vi "Test Acquisition API.vi"() -> ()   [LabVIEW 2026]
doc: "Acquisition API Tester.\n_____\nBased on DQMH Dev Tools: Project Template 7.1.2.1547."
uses:
  <vilib>/Utility/error.llb/DialogType.ctl
  Acquisition.lvlib
  Settings Editor/Settings Editor.lvlib
panel:
  in  "Show Diagram on Init":bool
  in  "Settings":bool
  out "last error":errorcluster
  out "Calibrated?":bool
  in  "Calibrate":bool
  out "Waveform Chart":waveform(dbl)[](graph)
  out "Acquiring?":bool
  in  "Stop Acquiring":bool
  out "HW ID":string
  in  "Start Acquiring":bool
  in  "Show Block Diagram":bool
  in  "Stop Module":bool
  in  "Start Module":bool
  in  "Hide Module Panel":bool
  in  "Show Module Panel":bool
  out "Status":string
  out "Module Running?":bool
  # "This VI tests the API for the Module."
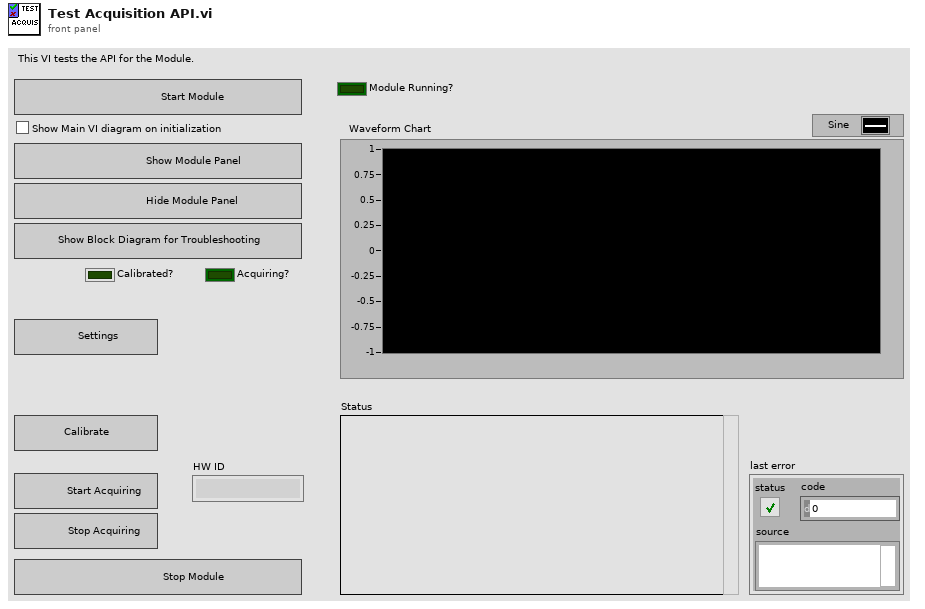
[diagram p1: front panel]
types:
  T1 = typedef "Acquisition.lvlib/Broadcast Events--cluster.ctl" = cluster{"Module Did Init":refnum<user-event>, "Status Updated":refnum<user-event>, "Error Reported":refnum<user-event>, "Module Did Stop":refnum<user-event>, "Update Module Execution Status":refnum<user-event>, "Acquisition Started":refnum<user-event>, "Acquisition Stopped":refnum<user-event>, "Data Updated":refnum<user-event>, "Device Calibrated":refnum<user-event>}
  T2 = typedef "DialogType.ctl" = u16
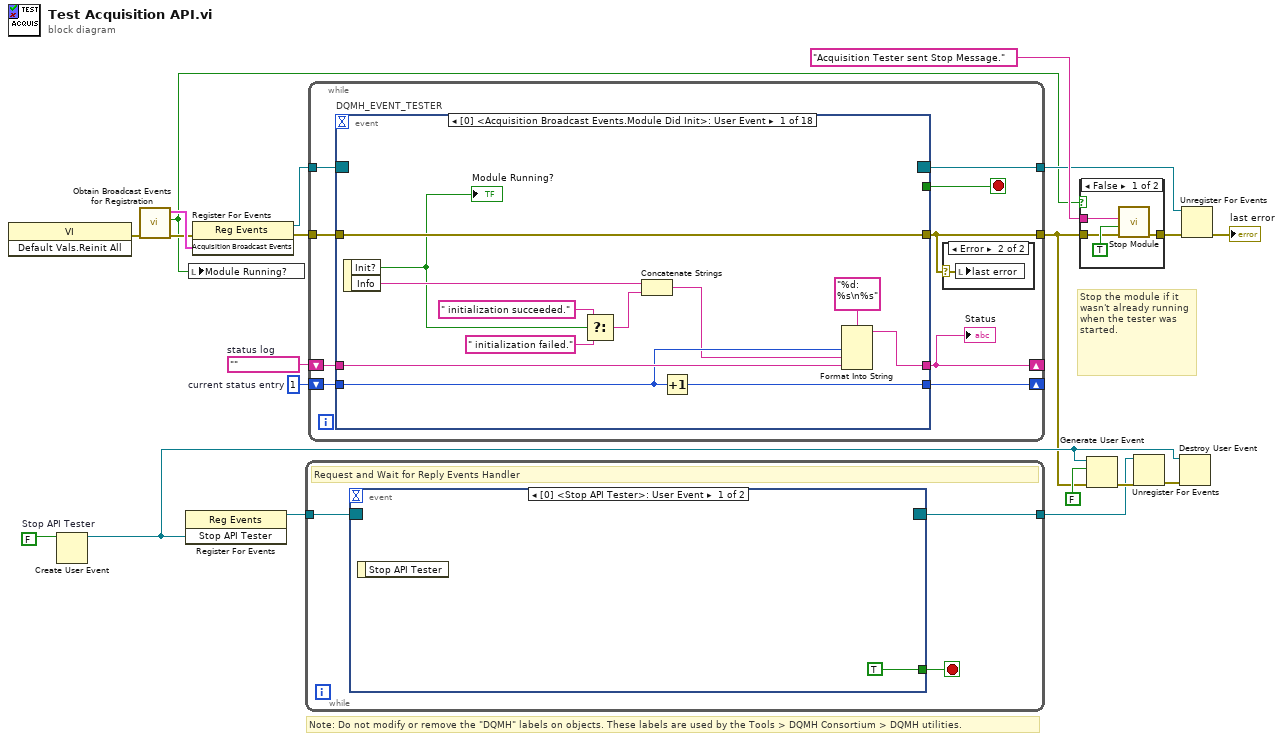
[diagram p0: block diagram]
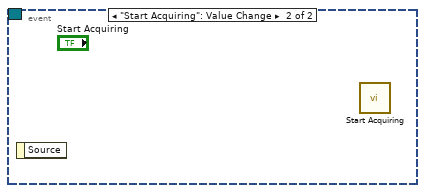
[diagram p2: hidden frame]
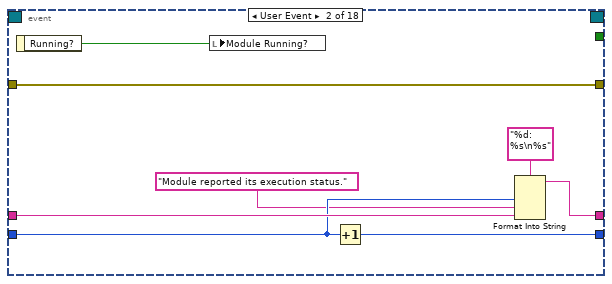
[diagram p4: hidden frame]
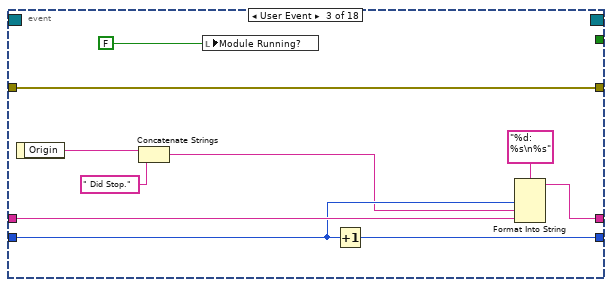
[diagram p5: hidden frame]
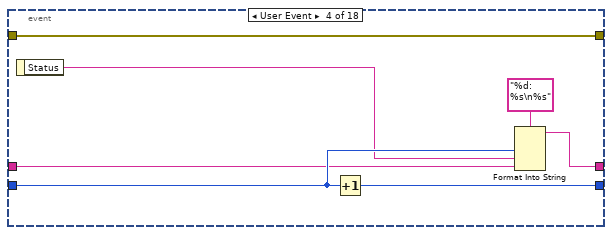
[diagram p6: hidden frame]
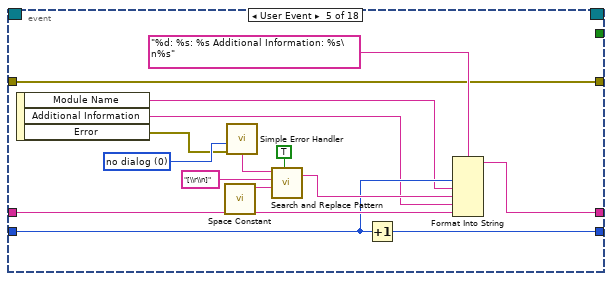
[diagram p7: hidden frame]
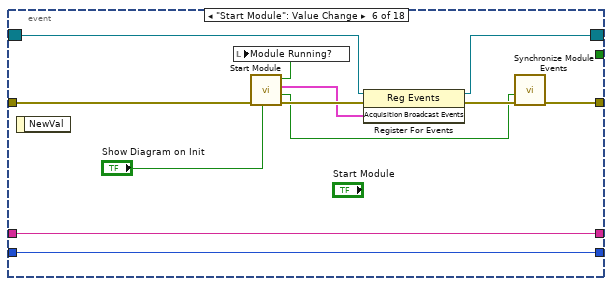
[diagram p8: hidden frame]
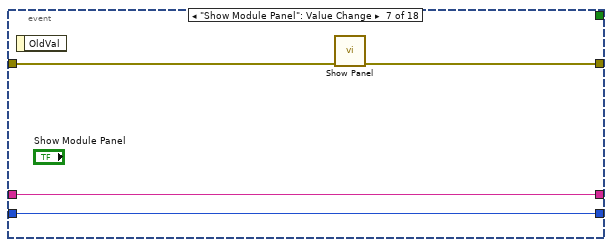
[diagram p9: hidden frame]
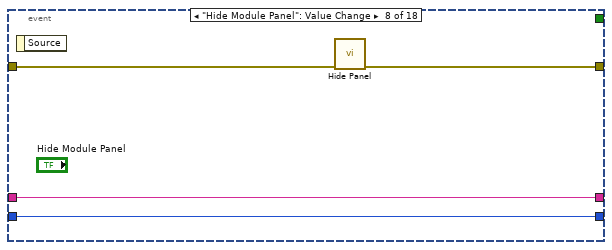
[diagram p10: hidden frame]
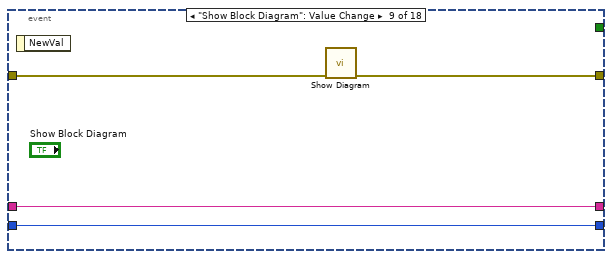
[diagram p11: hidden frame]
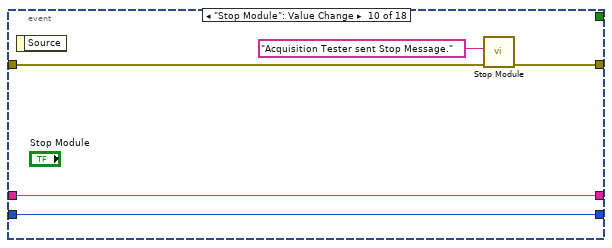
[diagram p12: hidden frame]
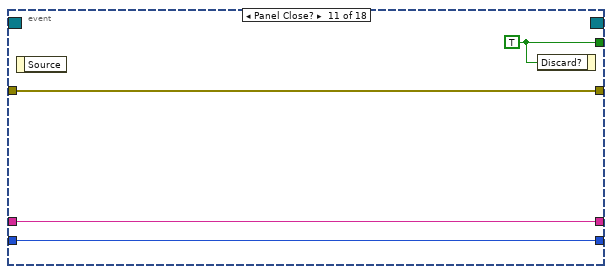
[diagram p13: hidden frame]
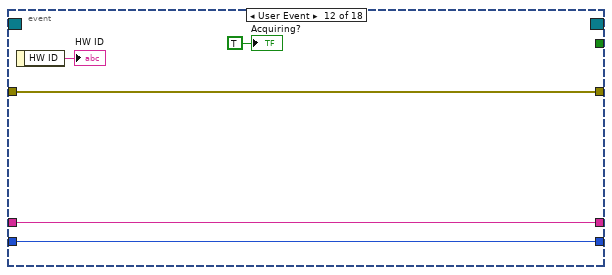
[diagram p14: hidden frame]
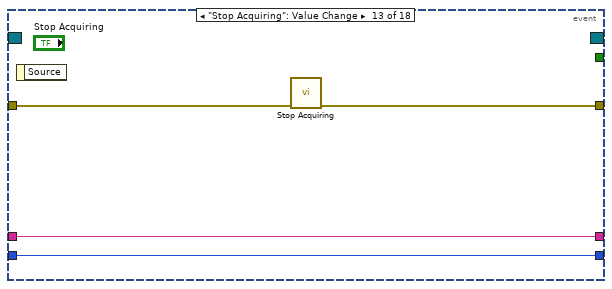
[diagram p15: hidden frame]
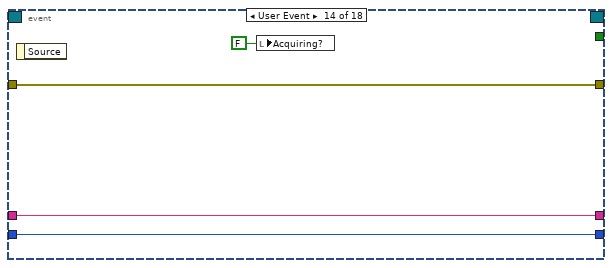
[diagram p16: hidden frame]
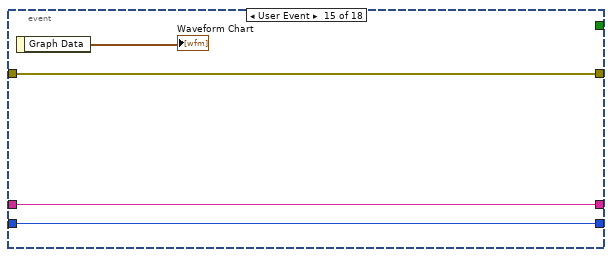
[diagram p17: hidden frame]
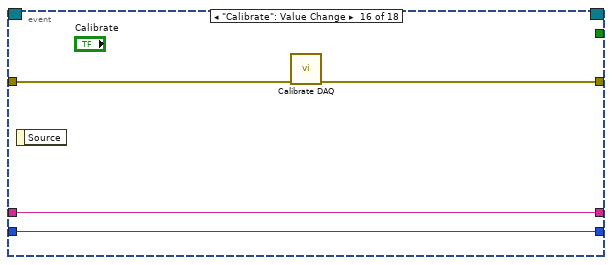
[diagram p18: hidden frame]
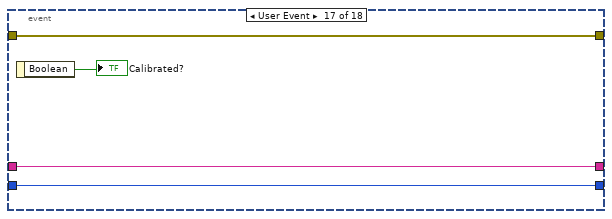
[diagram p19: hidden frame]
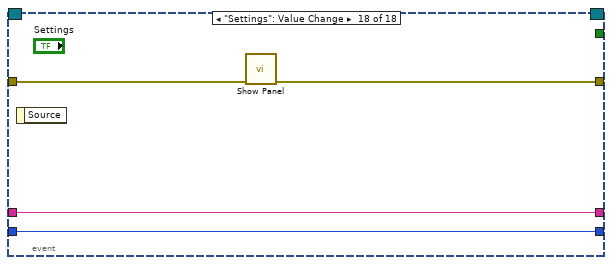
[diagram p20: hidden frame]
diagram:
  w10 = FALSE  # Stop API Tester
  w17 = 1  # current status entry
  w18 = ""  # status log
  # "Stop the module if it wasn't already running when the tester was started."
  # "Note: Do not modify or remove the \"DQMH\" labels on objects. These labels are used by the Tools > DQMH Consortium > DQMH utilities."
  n1 = invoke on="Invoke Node" class="VI" method="Default Vals.Reinit All"() -> (error out=w12:errorcluster)  [unwired: 3 in, 2 out]
  n2 = Create User Event(user event datatype=w10) -> (user event=w4:refnum<user-event>)  [unwired: 1 in, 1 out]
  n3 = call "Obtain Broadcast Events for Registration.vi"("error in"=w12) -> ("error out"=w11:errorcluster, "Already running?"=w3:bool, "Acquisition Broadcast Events"=w15:T1)  [unwired: 8 in]
  n4 = register-events(w4) -> (reference out=w9:refnum<event-registration>)  [unwired: 2 in, 1 out]
  n5 = local write "Module Running?"(w3) -> ()
  n6 = register-events(error in=w11, w15) -> (reference out=w14:refnum<event-registration>, error out=w16:errorcluster)  [unwired: 1 in]
  n7 = while {
    tunnel: w9 -> [w23]
    tunnel: [w21] -> w6
    stop <- w22 stop-if-true
    # "Request and Wait for Reply Events Handler"
    n8 = event shown="[0] <Stop API Tester>: User Event" {
      selector: w23 -> [_ _]
      dyn-events: [_ _] -> w21
      timeout: _ -> [_ _]
      tunnel: [TRUE _] -> w22
      event User Event {
        n9 = event-data() -> ()  [unwired: 1 in, 1 out]
      }
      event "Start Acquiring": Value Change {
        n10 = event-data() -> ()  [unwired: 1 in, 1 out]
        n11 = call "Start Acquiring.vi"() -> ()  [unwired: 9 in, 3 out]
      }
    }
  }
  n12 = while {
    tunnel: w14 -> [w33]
    tunnel: [w25] -> w2
    shift-right: [w29] -> _
    shift-left: w18 -> [w31]
    shift-right: [w30] -> _
    shift-left: w17 -> [w32]
    tunnel: w16 -> [w28]
    tunnel: [w27] -> w13
    stop <- w26 stop-if-true
    n13 = event "DQMH_EVENT_TESTER" shown="[0] <Acquisition Broadcast Events.Module Did Init>: User Event" {
      selector: w33 -> [_ _ _ _ _ w92 _ _ _ _ _ _ _ _ _ _ _ _]
      dyn-events: [_ _ _ _ _ w91 _ _ _ _ _ _ _ _ _ _ _ _] -> w27
      timeout: _ -> [_ _ _ _ _ _ _ _ _ _ _ _ _ _ _ _ _ _]
      tunnel: [_ _ _ _ _ _ _ _ _ _ w119 _ _ _ _ _ _ _] -> w26
      tunnel: [w46 w48 w55 w65 w75 w90 w102 w106 w107 w113 w116 w124 w125 w132 w136 w137 w144 w145] -> w25
      tunnel: w32 -> [w43 w52 w62 w68 w78 w95 w100 w104 w108 w114 w117 w122 w126 w130 w134 w138 w142 w147]
      tunnel: w31 -> [w44 w53 w63 w67 w79 w96 w101 w105 w109 w115 w118 w123 w127 w131 w135 w139 w143 w148]
      tunnel: [w41 w50 w60 w69 w76 w96 w101 w105 w109 w115 w118 w123 w127 w131 w135 w139 w143 w148] -> w29
      tunnel: [w42 w51 w61 w71 w77 w95 w100 w104 w108 w114 w117 w122 w126 w130 w134 w138 w142 w147] -> w30
      tunnel: w28 -> [w46 w48 w55 w65 w75 w89 w99 w103 w110 w111 w116 w124 w128 w132 w136 w140 w144 w146]
      event User Event {
        n14 = event-data() -> ("Init?"=w38:bool, "Info"=w40:string)  [unwired: 1 in]
        "Module Running?" <- w38
        n15 = Select(t=" initialization succeeded.", s=w38, f=" initialization failed.") -> (s? t:f=w35:string)
        n16 = Concatenate Strings(w40, w35) -> (w39:string)
        n17 = Increment(x=w43) -> (x+1=w42:i32)
        n18 = Format Into String(format string="%d: %s\n%s", w43, w39, w44) -> (resulting string=w41:string)  [unwired: 2 in, 1 out]
      }
      event User Event {
        n19 = event-data() -> ("Running?"=w47:bool)  [unwired: 1 in]
        n20 = local write "Module Running?"(w47) -> ()
        n21 = Increment(x=w52) -> (x+1=w51:i32)
        n22 = Format Into String(format string="%d: %s\n%s", w52, "Module reported its execution status.", w53) -> (resulting string=w50:string)  [unwired: 2 in, 1 out]
      }
      event User Event {
        n23 = event-data() -> ("Origin"=w59:string)  [unwired: 1 in]
        n24 = Concatenate Strings(w59, " Did Stop.") -> (w58:string)
        n25 = local write "Module Running?"(FALSE ("Module Did Init?")) -> ()
        n26 = Increment(x=w62) -> (x+1=w61:i32)
        n27 = Format Into String(format string="%d: %s\n%s", w62, w58, w63) -> (resulting string=w60:string)  [unwired: 2 in, 1 out]
      }
      event User Event {
        n28 = event-data() -> ("Status"=w66:string)  [unwired: 1 in]
        n29 = Increment(x=w68) -> (x+1=w71:i32)
        n30 = Format Into String(format string="%d: %s\n%s", w68, w66, w67) -> (resulting string=w69:string)  [unwired: 2 in, 1 out]
      }
      event User Event {
        w80 = T2 0 items=["no dialog", "OK message", "continue or stop message", "OK message + warnings", "continue/stop + warnings"] ("type of dialog (OK msg:1)")
        n31 = event-data() -> ("Module Name"=w74:string, "Additional Information"=w73:string, "Error"=w72:errorcluster)  [unwired: 1 in]
        n32 = call <vilib>:"Space Constant.vi"() -> ("String"=w84:string)
        n33 = call <vilib>:"Simple Error Handler.vi"("type of dialog (OK msg:1)"=w80, "error in (no error)"=w72) -> ("message"=w81:string)  [unwired: 3 in, 4 out]
        n34 = call <vilib>:"Search and Replace Pattern.vi"("string"=w81, "regular expression (\"\")"="[\\r\\n]" ("regular expression (\"\")"), "replace string (\"\")"=w84, "replace all? (F)"=TRUE ("replace all CR/LF with spaces")) -> ("result string"=w82:string)  [unwired: 1 in, 1 out]
        n35 = Increment(x=w78) -> (x+1=w77:i32)
        n36 = Format Into String(format string="%d: %s: %s Additional Information: %s\n%s", w78, w74, w82, w73, w79) -> (resulting string=w76:string)  [unwired: 2 in, 1 out]
      }
      event "Start Module": Value Change {
        n37 = event-data() -> ()  [unwired: 1 in, 1 out]
        n38 = call "Start Module.vi"("Show Main VI Diagram on Init (F)"="Show Diagram on Init", "error in"=w89) -> ("error out"=w97:errorcluster, "Wait for Event Sync?"=w94:bool, "Acquisition Broadcast Events"=w93:T1, "Module Was Already Running?"=w88:bool)  [unwired: 5 in, 1 out]
        n39 = local write "Module Running?"(w88) -> ()
        n40 = register-events(reference=w92, error in=w97, w93) -> (reference out=w91:refnum<event-registration>, error out=w98:errorcluster)
        n41 = call "Synchronize Module Events.vi"("error in"=w98, "Wait for Event Sync?"=w94) -> ("error out"=w90:errorcluster)  [unwired: 9 in]
      }
      event "Show Module Panel": Value Change {
        n42 = event-data() -> ()  [unwired: 1 in, 1 out]
        n43 = call "Show Panel.vi"("error in"=w99) -> ("error out"=w102:errorcluster)  [unwired: 10 in]
      }
      event "Hide Module Panel": Value Change {
        n44 = event-data() -> ()  [unwired: 1 in, 1 out]
        n45 = call "Hide Panel.vi"("error in"=w103) -> ("error out"=w106:errorcluster)  [unwired: 10 in]
      }
      event "Show Block Diagram": Value Change {
        n46 = event-data() -> ()  [unwired: 1 in, 1 out]
        n47 = call "Show Diagram.vi"("error in"=w110) -> ("error out"=w107:errorcluster)  [unwired: 10 in]
      }
      event "Stop Module": Value Change {
        n48 = event-data() -> ()  [unwired: 1 in, 1 out]
        n49 = call "Stop Module.vi"("error in"=w111, "Origin"="Acquisition Tester sent Stop Message.") -> ("error out"=w113:errorcluster)  [unwired: 9 in]
      }
      event Panel Close? {
        w119 = TRUE ("Discard?")
        n50 = event-data() -> ()  [unwired: 1 in, 1 out]
        n51 = event-data ("Event Filter Node")("Discard?"=w119) -> ()  [unwired: 1 in, 1 out]
      }
      event User Event {
        n52 = event-data() -> ("HW ID"=→"HW ID":string)  [unwired: 1 in]
        "Acquiring?" <- TRUE ("Acquiring?")
      }
      event "Stop Acquiring": Value Change {
        n53 = event-data() -> ()  [unwired: 1 in, 1 out]
        n54 = call "Stop Acquiring.vi"("error in"=w128) -> ("error out"=w125:errorcluster)  [unwired: 10 in]
      }
      event User Event {
        n55 = event-data() -> ()  [unwired: 1 in, 1 out]
        n56 = local write "Acquiring?"(FALSE ("Acquiring?")) -> ()
      }
      event User Event {
        n57 = event-data() -> ("Graph Data"=→"Waveform Chart":waveform(dbl)[])  [unwired: 1 in]
      }
      event "Calibrate": Value Change {
        n58 = event-data() -> ()  [unwired: 1 in, 1 out]
        n59 = call "Calibrate DAQ.vi"("error in"=w140) -> ("error out"=w137:errorcluster)  [unwired: 10 in]
      }
      event User Event {
        n60 = event-data() -> ("Boolean"=→"Calibrated?":bool)  [unwired: 1 in]
      }
      event "Settings": Value Change {
        n61 = event-data() -> ()  [unwired: 1 in, 1 out]
        n62 = call "Show Panel.vi"("error in"=w146) -> ("error out"=w145:errorcluster)  [unwired: 10 in]
      }
    }
    "Status" <- w29
    n63 = case shown="Error" w25 {
      selector: w25 -> [_ w34]
      frame No Error {
      }
      frame Error {
        n64 = local write "last error"(w34) -> ()
      }
    }
  }
  n65 = case shown="False" w3 {
    tunnel: [w152 w153] -> w20
    tunnel: "Acquisition Tester sent Stop Message." ("Origin") -> [w151 _]
    tunnel: w2 -> [w149 w153]
    frame False {
      n66 = call "Stop Module.vi"("error in"=w149, "Wait for Module to Stop? (F)"=TRUE ("Wait for Module to stop?"), "Origin"=w151) -> ("error out"=w152:errorcluster)  [unwired: 8 in]
    }
    frame True {
    }
  }
  n67 = Generate User Event(user event=w4, event data cluster=FALSE ("Stop API Tester"), error in=w2) -> (error out=w7:errorcluster)  [unwired: 1 in, 1 out]
  n68 = Unregister For Events(event registration refnum=w6, error in=w7) -> (error out=w5:errorcluster)
  n69 = Destroy User Event(user event=w4, error in=w5) -> ()  [unwired: 1 out]
  n70 = Unregister For Events(event registration refnum=w13, error in=w20) -> (error out=→"last error":errorcluster)
